vi "Operation Event Enable.vi"(0 "VISA resource name":refnum<visa-resource-name>, 5 "Operation Event Enable":T1, 11 "error in (no error)":errorcluster) -> (4 "VISA resource name out":refnum<visa-resource-name>, 15 "error out":errorcluster)   [LabVIEW 2018, in "XP Power PLS600.lvlib"]
doc: "Sets the value of the Operation Enable register. This register is a mask for enabling specific bits from the Operation Event register to set the operation summary bit (OPER) of the Status Byte register. The operation summary bit is the logical OR of all enabled Operation Event register bits.\n\nThe Operation Event Enable consists of the following 15 bits:\n\nBit 0: Calibrating\nBit 1: Setting\nBit 2: Ranging \nBit 3: Sweeping\nBit 4: Measuring\nBit 5: Waiting for Trigger \nBit 6: Waiting for Arm\nBit 7: Correcting\nBit 8: Output Enabled\nBit 9: Constant Voltage\nBit 10: Constant Current\nBit 11: Reserved\nBit 12: Reserved\nBit 13: Instrument Summary\nBit 14: Program Running\nBit 15: Reserved"
uses:
  XP Power PLS600.lvlib
panel:
  # "Bit 0:  Calibrating\nBit 1:  Setting\nBit 2:  Ranging\t\nBit 3:  Sweeping\nBit 4:\t\tMeasuring\nBit 5:  Waiting for Trigger\t\nBit 6:  Waiting for Arm\nBit 7:  Correcting\nBit 8:  Output Enabled\nBit 9:  Constant Voltage\nBit 10:  Constant Current\nBit 11:  Reserved\nBit 12:  Reserved\nBit 13:  Instrument Summary\nBit 14:  Program Running\nBit 15:  Reserved"
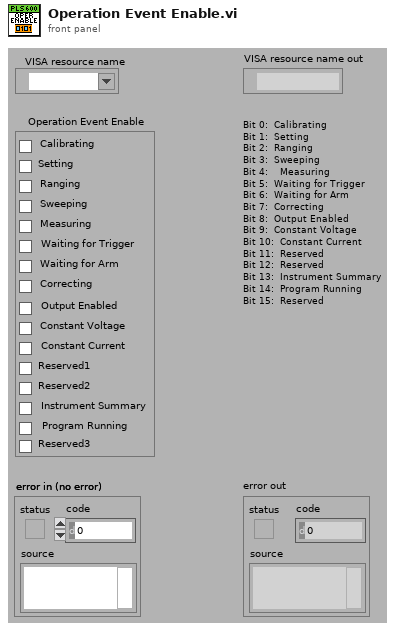
[diagram p1: front panel]
types:
  T1 = cluster{"Calibrating":bool, "Setting":bool, "Ranging":bool, "Sweeping":bool, "Measuring":bool, "Waiting for Trigger":bool, "Waiting for Arm":bool, "Correcting":bool, "Output Enabled":bool, "Constant Voltage":bool, "Constant Current":bool, "Reserved1":bool, "Reserved2":bool, "Instrument Summary":bool, "Program Running":bool, "Reserved3":bool}
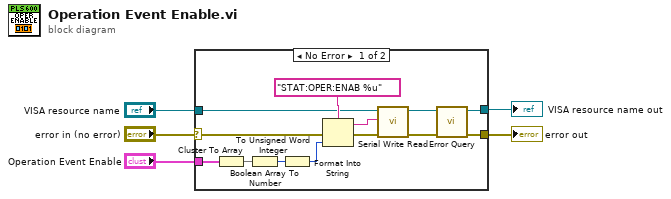
[diagram p0: block diagram]
diagram:
  n1 = case shown="No Error" "error in (no error)" {
    selector: "error in (no error)" -> [w18 w20]
    tunnel: "VISA resource name" -> [w7 w19]
    tunnel: [w8 w19] -> w5
    tunnel: [w9 w20] -> w4
    tunnel: "Operation Event Enable" -> [w15 _]
    frame No Error {
      n2 = Cluster To Array(cluster=w15) -> (array=w16:bool[])
      n3 = Boolean Array To Number(Boolean array=w16) -> (number=w14:u32)
      n4 = To Unsigned Word Integer(number=w14) -> (unsigned 16bit integer=w13:u16)
      n5 = Format Into String(format string="STAT:OPER:ENAB %u" ("Command to Send"), error in=w18, w13) -> (resulting string=w6:string, error out=w10:errorcluster)  [unwired: 1 in]
      n6 = call "Serial Write Read.vi"("error in (no error)"=w10, "Write Buffer"=w6, "VISA resource name"=w7) -> ("error out"=w12:errorcluster, "VISA resource name out"=w11:refnum<visa-resource-name>)  [unwired: 6 in, 1 out]
      n7 = call "Error Query.vi"("error in (no error)"=w12, "VISA resource name"=w11) -> ("error out"=w9:errorcluster, "VISA resource name out"=w8:refnum<visa-resource-name>)  [unwired: 6 in, 2 out]
    }
    frame Error {
    }
  }
  "error out" <- w4
  "VISA resource name out" <- w5
